vi "pipx40 Set Channel Pattern.vi"(4 "error in (no error)":errorcluster, 5 "pattern":u32[](array[numeric]), 6 "subunit number":u32=1, 7 "instrument handle":refnum<visa-resource-name>) -> (0 "error out":errorcluster, 2 "status":i32 format="%.0x", 3 "instrument handle out":refnum<visa-resource-name>)   [LabVIEW 2011]
doc: "Sets all channels of an output sub-unit using a supplied bit-pattern."
uses:
  pipx40_32.dll
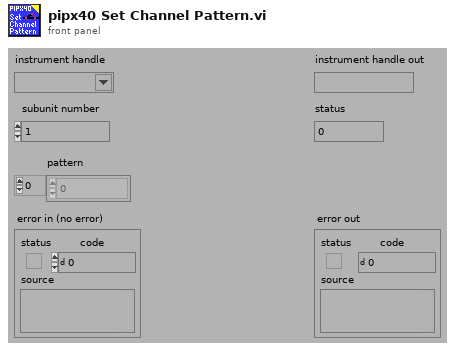
[diagram p1: front panel]
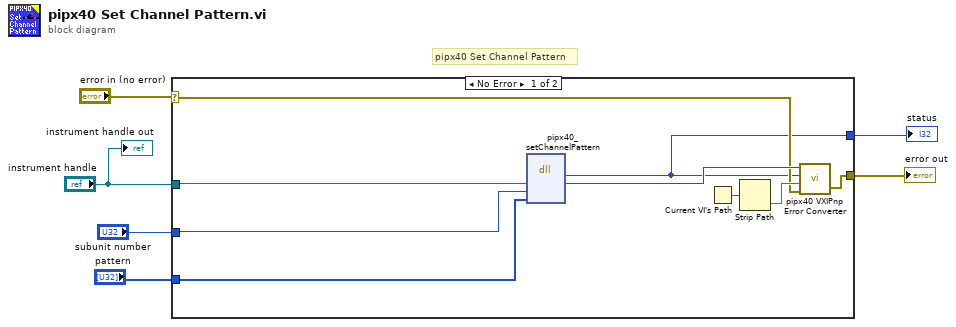
[diagram p0: block diagram]
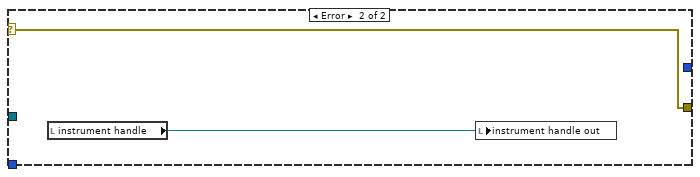
[diagram p2: hidden frame]
diagram:
  # "pipx40 Set Channel Pattern"
  n1 = case shown="No Error" "error in (no error)" {
    selector: "error in (no error)" -> [w11 w16]
    tunnel: [w12 w16] -> w6
    tunnel: [w7 _] -> w4
    tunnel: "pattern" -> [w10 _]
    tunnel: "subunit number" -> [w9 _]
    tunnel: "instrument handle" -> [w8 _]
    frame No Error {
      n2 = dll-call lib="pipx40_32.dll" fn="pipx40_setChannelPattern" label="pipx40 Set Channel Pattern"("instrument handle"=w8, "subunit number"=w9, "pattern"=w10) -> ("status"=w7:i32, "instrument handle"=w15:u32)  [unwired: 5 in, 2 out]
      n3 = Current VI's Path() -> (path=w14:path)
      n4 = Strip Path(path=w14) -> (name=w13:string)  [unwired: 1 out]
      n5 = call "pipx40 VXIPnp Error Converter.vi"("error in (no error)"=w11, "name of VI (\"\")"=w13, "VXIPnp error code (0)"=w7, "instrument handle"=w15) -> ("error out"=w12:errorcluster)  [unwired: 1 out]
    }
    frame Error {
      n6 = local read "instrument handle"() -> (w17:refnum<visa-resource-name>)
      n7 = local write "instrument handle out"(w17) -> ()
    }
  }
  "error out" <- w6
  "status" <- w4
  "instrument handle out" <- "instrument handle"
